vi "ClimbBegin.vi"(8 "error in (no error)":errorcluster) -> (0 "error out":errorcluster)   [LabVIEW 2023]
uses:
  <vilib>/Rock Robotics/WPI/ThirdParty/REV Robotics/REVLib/Typedef/Spark MAX Idle Mode.ctl
  <vilib>/Rock Robotics/WPI/ThirdParty/REV Robotics/REVLib/Typedef/Spark MAX Limit Switch Polarity.ctl
  <vilib>/Rock Robotics/WPI/ThirdParty/REV Robotics/REVLib/SubVI/Public/SPARK Open Brushless.vi
  <vilib>/Rock Robotics/WPI/ThirdParty/REV Robotics/REVLib/SubVI/Public/SPARK Configure Encoder Conversion Factors.vi
  <vilib>/Rock Robotics/WPI/ThirdParty/REV Robotics/REVLib/SubVI/Public/SPARK Configure Power Smart Current Limit.vi
  <vilib>/Rock Robotics/WPI/ThirdParty/REV Robotics/REVLib/SubVI/Public/SPARK Configure Basic Idle Mode.vi
  <vilib>/Rock Robotics/WPI/ThirdParty/REV Robotics/REVLib/SubVI/Public/SPARK Configure Limit Switch Reverse.vi
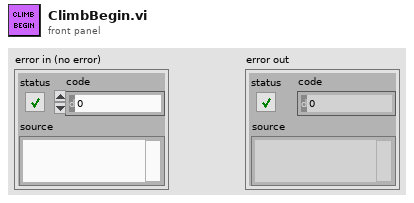
[diagram p1: front panel]
types:
  T1 = typedef "Spark MAX Idle Mode.ctl" = enum16{"Coast", "Brake"}
  T2 = typedef "Spark MAX Limit Switch Polarity.ctl" = enum16{"Normally Open", "Normally Closed"}
  T3 = typedef "WPI_MotorControlDeviceRef.ctl" = cluster{"DeviceStatus":errorcluster, "Type":T4, "PWM":cluster{"PWM Channel":T5, "DeadBand":T6}, "CAN":cluster{"Device Number":u8, "SetOutput VI Ref":variant, "GetOutput VI Ref":variant, "Enable VI Ref":variant, "Disable VI Ref":variant, "Data":variant}, "Invert":bool, "DIO PWM":cluster{"PWM \"Enable\" Channel":T5, "DIOChannel":T7, "PWM Rate":dbl}}
  T4 = typedef "WPI_MotorControlType.ctl" = enum16{"PWM", "CAN", "DIO PWM"}
  T5 = typedef "FPGA_DIOPWMChannel.ctl" = enum8{"PWM 0", "PWM 1", "PWM 2", "PWM 3", "PWM 4", "PWM 5", "PWM 6", "PWM 7", "PWM 8", "PWM 9", "PWM MXP 0", "PWM MXP 1", "PWM MXP 2", "PWM MXP 3", "PWM MXP 4", "PWM MXP 5", "PWM MXP 6", "PWM MXP 7", "PWM MXP 8", "PWM MXP 9", "Invalid"}
  T6 = typedef "WPI_PWMDeadband.ctl" = cluster{"Name":string, "maxPositivePwm":i32, "minPositivePwm":i32, "centerPwm":i32, "maxNegativePwm":i32, "minNegativePwm":i32, "angularRange":u16}
  T7 = typedef "FPGA_DIOChannel.ctl" = enum8{"DIO 0", "DIO 1", "DIO 2", "DIO 3", "DIO 4", "DIO 5", "DIO 6", "DIO 7", "DIO 8", "DIO 9", "DIO MXP 0", "DIO MXP 1", "DIO MXP 2", "DIO MXP 3", "DIO MXP 4", "DIO MXP 5", "DIO MXP 6", "DIO MXP 7", "DIO MXP 8", "DIO MXP 9", "DIO MXP 10", "DIO MXP 11", "DIO MXP 12", "DIO MXP 13", "DIO MXP 14", "DIO MXP 15", "SPI Port CS1", "SPI Port CS2", "SPI Port CS3", "SPI Port MISO", "SPI Port MOSI", "Invalid"}
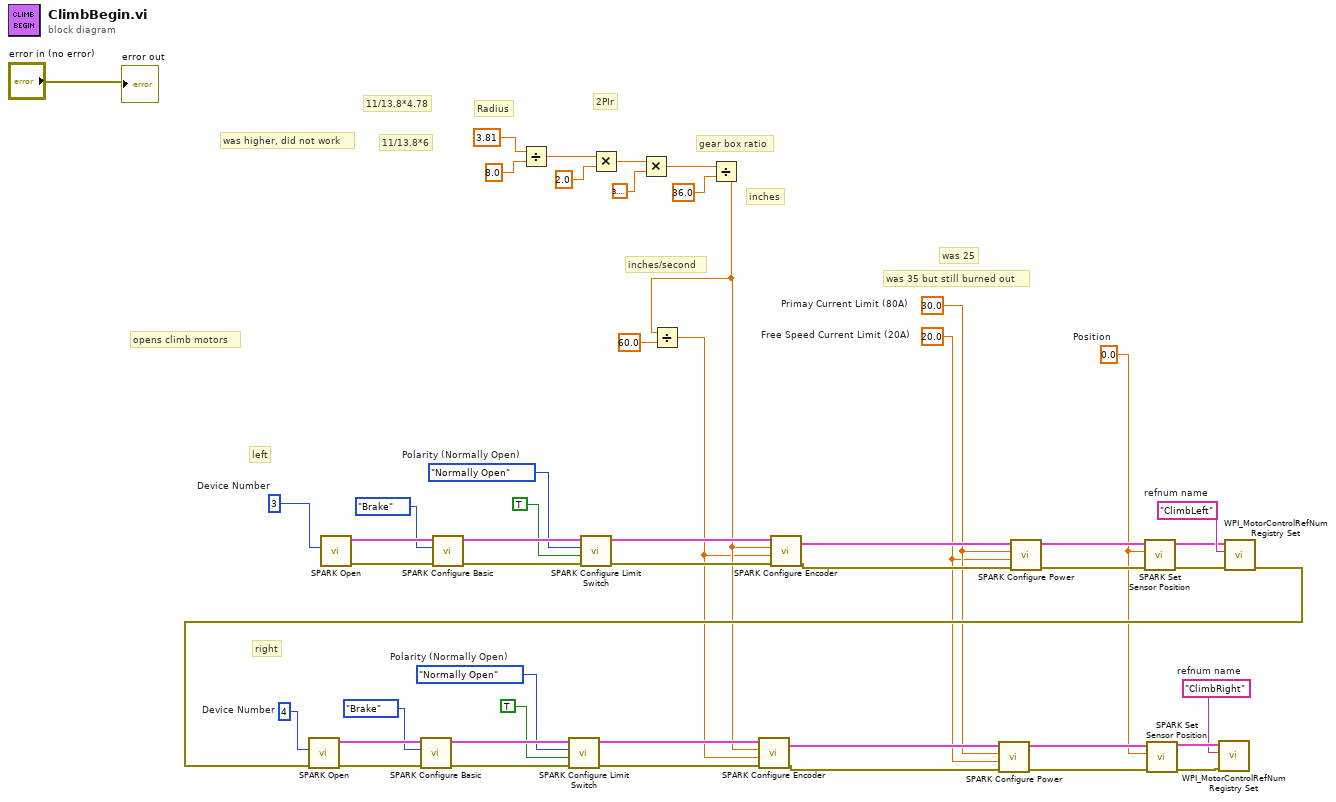
[diagram p0: block diagram]
diagram:
  w14 = Spark_MAX_Limit_Switch_Polarity."Normally Open"  # Polarity (Normally Open)
  w3 = 0.0  # Position
  w4 = 20.0  # Free Speed Current Limit (20A)
  w5 = 30.0  # Primay Current Limit (80A)
  w29 = Spark_MAX_Limit_Switch_Polarity."Normally Open"  # Polarity (Normally Open)
  w48 = "ClimbRight"  # refnum name
  w49 = "ClimbLeft"  # refnum name
  w25 = u8 4  # Device Number
  w8 = u8 3  # Device Number
  # "was 35 but still burned out"
  # "11/13.8*4.78"
  # "was higher, did not work"
  # "11/13.8*6"
  # "was 25"
  # "inches/second"
  # "inches"
  # "gear box ratio"
  # "2PIr"
  # "Radius"
  # "opens climb motors"
  # "right"
  # "left"
  n1 = call-poly <vilib>:"SPARK Open.vi"("Device Number"=w8) -> ("error out"=w20:errorcluster, "MotorControlDeviceRef"=w21:T3)  [unwired: 9 in]
  n2 = call-poly <vilib>:"SPARK Configure Basic.vi"("error in (no error)"=w20, "Idle Mode"=Spark_MAX_Idle_Mode."Brake", "MotorControlDeviceRef in"=w21) -> ("error out"=w15:errorcluster, "MotorControlDeviceRef out"=w16:T3)  [unwired: 7 in]
  n3 = Divide(x=3.81, y=8.0) -> (x/y=w44:dbl)
  n4 = call-poly <vilib>:"SPARK Configure Limit Switch.vi"("error in"=w15, "Enabled? (T)"=TRUE, "Polarity (Normally Open)"=w14, "MotorControlDeviceRef in"=w16) -> ("error out"=w11:errorcluster, "MotorControlDeviceRef out"=w12:T3)  [unwired: 6 in]
  n5 = Multiply(x=w44, y=2.0) -> (x*y=w42:dbl)
  n6 = Multiply(x=w42, y=3.141592653589793) -> (x*y=w40:dbl)
  n7 = Divide(x=w40, y=36.0) -> (x/y=w7:dbl)
  n8 = Divide(x=w7, y=60.0) -> (x/y=w6:dbl)
  n9 = call-poly <vilib>:"SPARK Configure Encoder.vi"("error in"=w11, "Velocity Conversion Factor"=w6, "Position Conversion Factor"=w7, "MotorControlDeviceRef in"=w12) -> ("error out"=w17:errorcluster, "MotorControlDeviceRef out"=w18:T3)  [unwired: 6 in]
  n10 = call-poly <vilib>:"SPARK Configure Power.vi"("error in (no error)"=w17, "Free Speed Current Limit (20A)"=w4, "Primay Current Limit (80A)"=w5, "MotorControlDeviceRef in"=w18) -> ("error out"=w9:errorcluster, "MotorControlDeviceRef out"=w10:T3)  [unwired: 6 in]
  n11 = call <vilib>:"SPARK Set Sensor Position.vi"("error in"=w9, "Position"=w3, "MotorControlDeviceRef"=w10) -> ("error out"=w1:errorcluster, "MotorControlDeviceRef"=w2:T3)  [unwired: 7 in]
  n12 = call <vilib>:"WPI_MotorControlRefNum Registry Set.vi"("error in (no error)"=w1, "refnum name"=w49, "MotorControlDevRef"=w2) -> ("error out"=w24:errorcluster)  [unwired: 7 in, 1 out]
  n13 = call-poly <vilib>:"SPARK Open.vi"("error in (no error)"=w24, "Device Number"=w25) -> ("error out"=w35:errorcluster, "MotorControlDeviceRef"=w36:T3)  [unwired: 8 in]
  n14 = call-poly <vilib>:"SPARK Configure Basic.vi"("error in (no error)"=w35, "Idle Mode"=Spark_MAX_Idle_Mode."Brake", "MotorControlDeviceRef in"=w36) -> ("error out"=w30:errorcluster, "MotorControlDeviceRef out"=w31:T3)  [unwired: 7 in]
  n15 = call-poly <vilib>:"SPARK Configure Limit Switch.vi"("error in"=w30, "Enabled? (T)"=TRUE, "Polarity (Normally Open)"=w29, "MotorControlDeviceRef in"=w31) -> ("error out"=w26:errorcluster, "MotorControlDeviceRef out"=w27:T3)  [unwired: 6 in]
  n16 = call-poly <vilib>:"SPARK Configure Encoder.vi"("error in"=w26, "Velocity Conversion Factor"=w6, "Position Conversion Factor"=w7, "MotorControlDeviceRef in"=w27) -> ("error out"=w32:errorcluster, "MotorControlDeviceRef out"=w33:T3)  [unwired: 6 in]
  n17 = call-poly <vilib>:"SPARK Configure Power.vi"("error in (no error)"=w32, "Free Speed Current Limit (20A)"=w4, "Primay Current Limit (80A)"=w5, "MotorControlDeviceRef in"=w33) -> ("error out"=w22:errorcluster, "MotorControlDeviceRef out"=w23:T3)  [unwired: 6 in]
  n18 = call <vilib>:"SPARK Set Sensor Position.vi"("error in"=w22, "Position"=w3, "MotorControlDeviceRef"=w23) -> ("error out"=w47:errorcluster, "MotorControlDeviceRef"=w50:T3)  [unwired: 7 in]
  n19 = call <vilib>:"WPI_MotorControlRefNum Registry Set.vi"("error in (no error)"=w47, "refnum name"=w48, "MotorControlDevRef"=w50) -> ()  [unwired: 7 in, 2 out]
  "error out" <- "error in (no error)"
